vi "DigitalWrite.vi"(0 "State":u16(ring) items=["LO", "HI"], 2 "Info In":cluster{"Numeric":u8}, 3 "Port":u8) -> (1 "Reply":string, 4 "Info Out":cluster{"Numeric":u8})   [LabVIEW 2014]
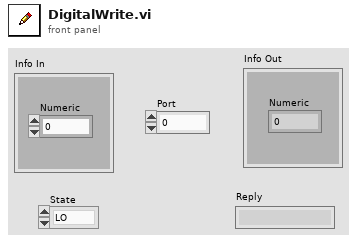
[diagram p1: front panel]
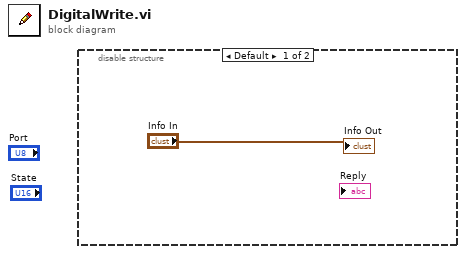
[diagram p0: block diagram]
diagram:
  n1 = disable-structure shown="Default" {
    frame condition #0 (active) {
      "Info Out" <- "Info In"
    }
    frame condition #1 {
    }
  }
